vi "Sql Cammand.vi"() -> ()   [LabVIEW 2015]
uses:
  <vilib>/addons/database/Connection.llb/DB Tools Open Connec (String).vi
  <vilib>/addons/database/Connection.llb/Conn Execute.vi
  <vilib>/addons/database/NI_Database_API.lvlib
panel:
  in  "Listbox":i32(listbox)
  in  "Enum":T1(ring)
  out "error out":errorcluster
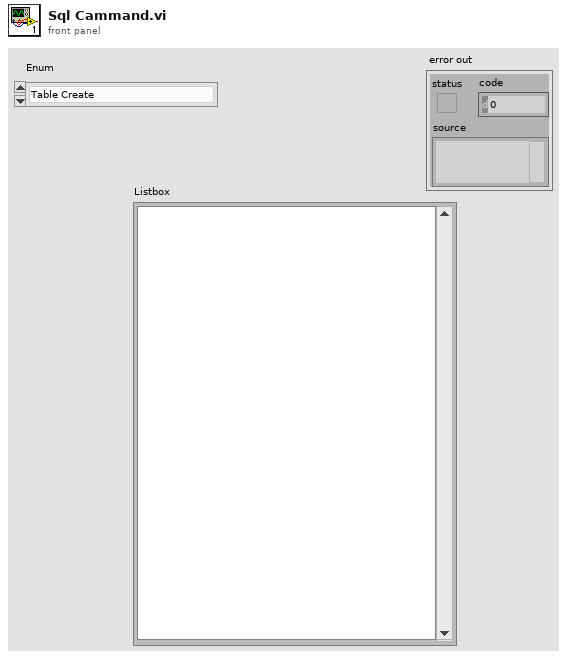
[diagram p1: front panel]
types:
  T1 = enum16{"Table Create", "SQL Backup", "Data Search", "Table Delete"}
  T2 = typedef "NI_Database_API.lvlib/Conn ObjectReference.ctl" = refnum<k1>
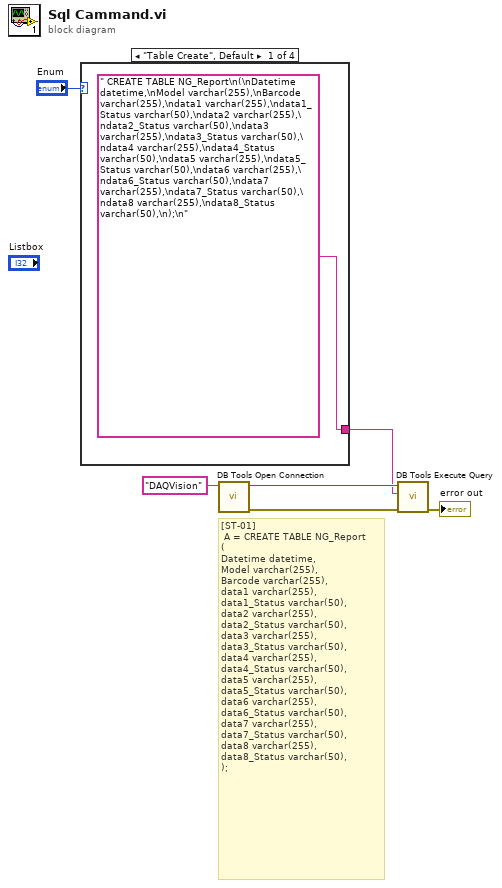
[diagram p0: block diagram]
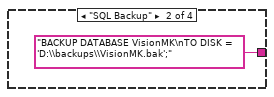
[diagram p2: hidden frame]
diagram:
  # "[ST-01]\n A = CREATE TABLE NG_Report\n(\nDatetime datetime,\nModel varchar(255),\nBarcode varchar(255),\ndata1 varchar(255),\ndata1_Status varchar(50),\ndata2 varchar(255),\ndata2_Status varchar(50),\ndata3 varchar(255),\ndata3_Status varchar(50),\ndata4 varchar(255),\ndata4_Status varchar(50),\ndata5 varchar(255),\ndata5_Status varchar(50),\ndata6 varchar(255),\ndata6_Status varchar(50),\ndata7 varchar(255),\ndata7_Status varchar(50),\ndata8 varchar(255),\ndata8_Status varchar(50),\n);"
  n1 = case shown="\"Table Create\", Default" "Enum" {
    tunnel: [" CREATE TABLE NG_Report\n(\nDatetime datetime,\nModel varchar(255),\nBarcode varchar(255),\ndata1 varchar(255),\ndata1_Status varchar(50),\ndata2 varchar(255),\ndata2_Status varchar(50),\ndata3 varchar(255),\ndata3_Status varchar(50),\ndata4 varchar(255),\ndata4_Status varchar(50),\ndata5 varchar(255),\ndata5_Status varchar(50),\ndata6 varchar(255),\ndata6_Status varchar(50),\ndata7 varchar(255),\ndata7_Status varchar(50),\ndata8 varchar(255),\ndata8_Status varchar(50),\n);\n" ("SQL query") "BACKUP DATABASE VisionMK\nTO DISK = 'D:\\backups\\VisionMK.bak';" ("SQL query") _ _] -> w1
    frame "Table Create", Default {
    }
    frame "SQL Backup" {
    }
    frame "Data Search" {
    }
    frame "Table Delete" {
    }
  }
  n2 = call-poly <vilib>:"DB Tools Open Connection.vi"("connection information"="DAQVision" ("password")) -> ("error out"=w5:errorcluster, "connection reference"=w6:T2)  [unwired: 7 in]
  n3 = call-poly <vilib>:"DB Tools Execute Query.vi"("error in (no error)"=w5, "SQL query"=w1, "connection reference"=w6) -> ("error out"=→"error out":errorcluster)  [unwired: 5 in, 1 out]
